vi "BRig_Host__global__stopHost.vi"() -> ()   [LabVIEW 2014]
panel:
  out "global_stopHost":bool
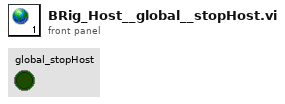
[diagram p1: front panel]
diagram:
